vi "configure.vi"(8 "error in (no error)":errorcluster, 11 "GenericPlugin in":refnum<class "LightSourceMH110125Tsunami.lvclass">) -> (0 "error out":errorcluster, 3 "GenericPlugin out":refnum<class "LightSourceMH110125Tsunami.lvclass">)   [LabVIEW 2010, in "LightSourceMH110125Tsunami.lvclass"]
doc: "The dynamic dispatch version of this VI loads and displays the configuration file associated with the plug-in object. The user modify and save the configuration data."
uses:
  LightSourceMH110125Tsunami.lvclass
  LightSourceMH110125Tsunami.lvclass/LightSourceMH110125Tsunami.ctl
  common/classes/GenericComponent/GenericComponent/GenericComponent.lvclass
panel:
  in  "Serial port":refnum<visa-resource-name>
  in  "Switch laser on at start up?":bool caption="Switch laser on\nat start up?"
  in  "Maximal power":dbl[unit]=800.0
  in  "Read delay (ms)":u32=50
  in  "Data bits":u16=8
  in  "Baud rate":u32=9600
  in  "Parity (0:none)":enum16{"None", "Odd", "Even", "Mark", "Space"}(ring)
  in  "Stop bits":u16(ring)=10 items=["1.0"=10, "1.5"=15, "2.0"=20]
  in  "Flow control":u16(ring)=1 items=["None"=0, "XON/XOFF"=1, "RTS/CTS"=2, "DTR/DSR"=4]
  in  "cancel":bool
  in  "save":bool
  out "Configuration":string
  # "Configure MH110117Tsunami"
  # "laser settings"
  # "port settings"
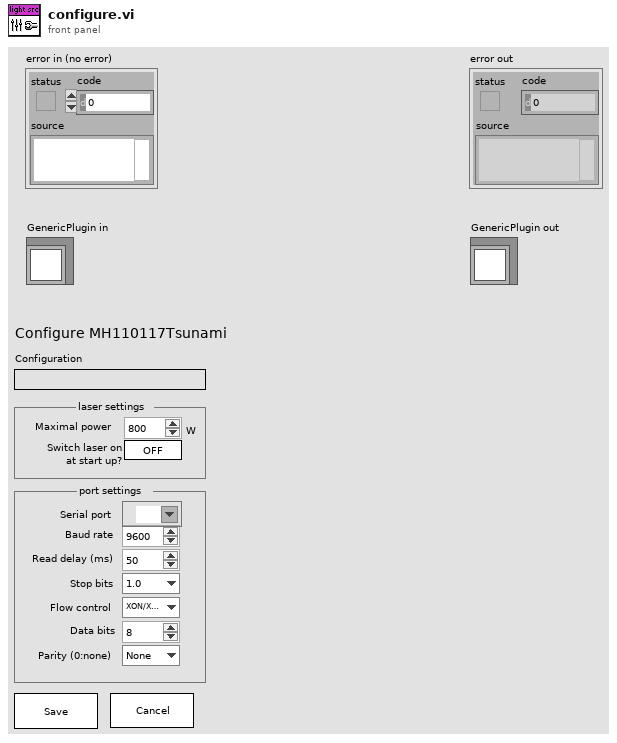
[diagram p1: front panel]
types:
  T1 = typedef "LightSourceMH110125Tsunami.lvclass/config_data_cluster.ctl" = cluster{"hardware settings":cluster{"comm port":string, "switch laser on?":bool, "open shutter?":bool, "max power":dbl[unit], "delay before read (ms)":u32, "flow control":u16, "stop bits":u16, "data bits":u16, "baud rate":u32, "parity (0:none)":enum16{"None", "Odd", "Even", "Mark", "Space"}}}
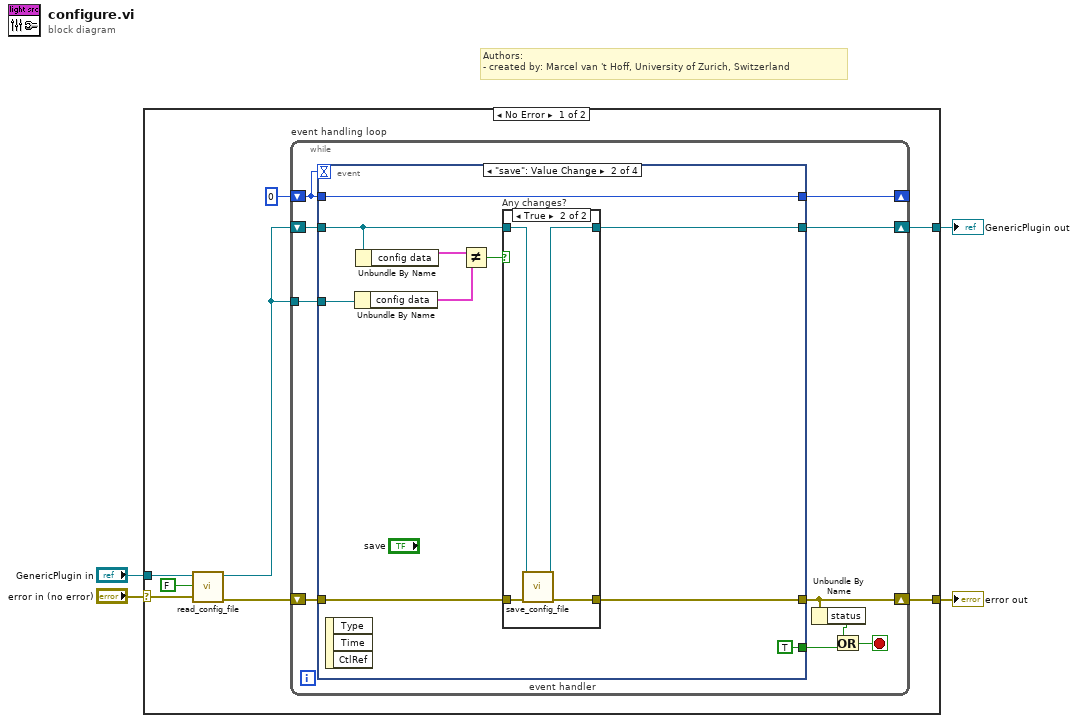
[diagram p0: block diagram]
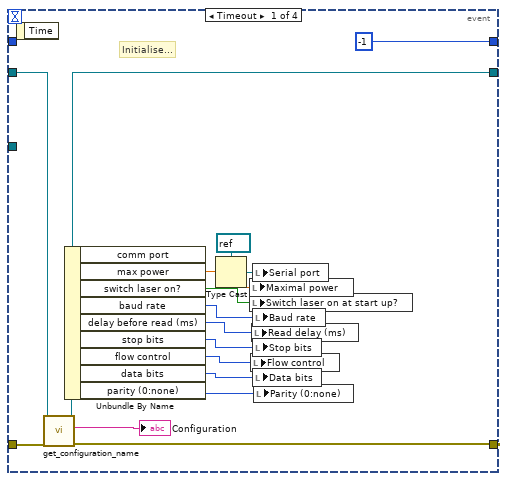
[diagram p2: hidden frame]
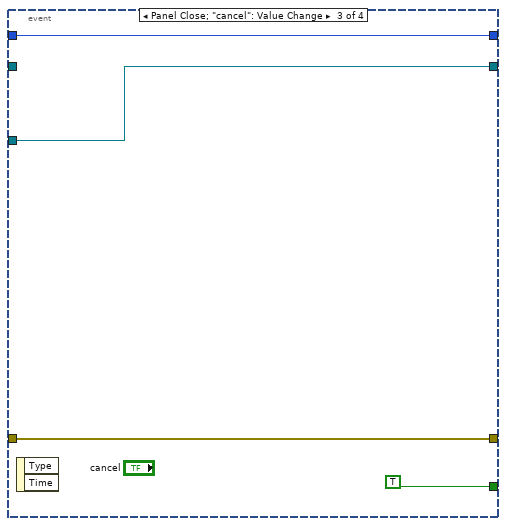
[diagram p4: hidden frame]
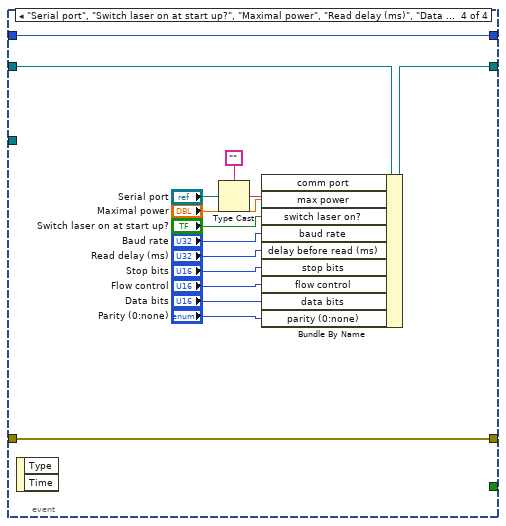
[diagram p5: hidden frame]
diagram:
  # "Authors: \n- created by: Marcel van 't Hoff, University of Zurich, Switzerland"
  n1 = case shown="No Error" "error in (no error)" {
    selector: "error in (no error)" -> [w10 w75]
    tunnel: "GenericPlugin in" -> [w8 w76]
    tunnel: [w12 w76] -> w1
    tunnel: [w11 w75] -> w2
    frame No Error {
      n2 = call-dynamic "read_config_file.vi"("error in (no error)"=w10, "force load?"=FALSE, "GenericPlugin in"=w8) -> ("error out"=w6:errorcluster, "GenericPlugin out"=w5:refnum<class "LightSourceMH110125Tsunami.lvclass">)  [unwired: 7 in]
      n3 = while "event handling loop" {
        shift-right: [w17] -> w11
        shift-left: w6 -> [w22]
        shift-right: [w20] -> w12
        shift-left: w5 -> [w21]
        shift-right: [w18] -> _
        shift-left: 0 -> [w19]
        tunnel: w5 -> [w13]
        stop <- w14 stop-if-true
        n4 = event "event handler" shown="[1] \"save\": Value Change" {
          selector: _ -> [_ _ _ _]
          dyn-events: _ -> [_ _ _ _]
          timeout: w19 -> [_ _ _ _]
          tunnel: w22 -> [w28 w47 w59 w60]
          tunnel: w21 -> [w25 w46 _ w62]
          tunnel: [w24 w43 w56 w61] -> w20
          tunnel: [w26 w44 w59 w60] -> w17
          tunnel: [_ TRUE TRUE _] -> w15
          tunnel: [-1 w48 w57 w74] -> w18
          tunnel: w19 -> [_ w48 w57 w74]
          tunnel: w13 -> [_ w41 w56 _]
          event Timeout {
            # "Initialise..."
            n5 = event-data() -> ()  [unwired: 1 in, 1 out]
            n6 = call "get_configuration_name.vi"("error in (no error)"=w28, "GenericPlugin.lvclass in"=w25) -> ("error out"=w26:errorcluster, "configuration name"=→"Configuration":string, "GenericPlugin.lvclass out"=w24:refnum<class "LightSourceMH110125Tsunami.lvclass">)  [unwired: 7 in]
            n7 = Unbundle By Name(w24) -> ("comm port"=w31:string, "max power"=w32:dbl[unit], "switch laser on?"=w33:bool, "baud rate"=w34:u32, "delay before read (ms)"=w35:u32, "stop bits"=w36:u16, "flow control"=w37:u16, "data bits"=w38:u16, "parity (0:none)"=w23:enum16{"None", "Odd", "Even", "Mark", "Space"})
            n8 = Type Cast(type=refnum<visa-resource-name> refnum ("Serial port"), x=w31) -> (*(type *) &x=w30:refnum<visa-resource-name>)
            n9 = local write "Maximal power"(w32) -> ()
            n10 = local write "Switch laser on at start up?"(w33) -> ()
            n11 = local write "Flow control"(w37) -> ()
            n12 = local write "Read delay (ms)"(w35) -> ()
            n13 = local write "Serial port"(w30) -> ()
            n14 = local write "Baud rate"(w34) -> ()
            n15 = local write "Stop bits"(w36) -> ()
            n16 = local write "Data bits"(w38) -> ()
            n17 = local write "Parity (0:none)"(w23) -> ()
          }
          event "save": Value Change {
            n18 = event-data() -> ()  [unwired: 1 in, 3 out]
            n19 = Unbundle By Name(w41) -> ("config data"=w40:T1)
            n20 = Unbundle By Name(w46) -> ("config data"=w42:T1)
            n21 = Not Equal?(x=w42, y=w40) -> (x != y?=w45:bool)
            n22 = case "Any changes?" shown="True" w45 {
              tunnel: w47 -> [w51 w54]
              tunnel: [w51 w53] -> w44
              tunnel: w46 -> [w50 w55]
              tunnel: [w50 w52] -> w43
              frame False {
              }
              frame True {
                n23 = call-dynamic "save_config_file.vi"("error in (no error)"=w54, "GenericPlugin in"=w55) -> ("error out"=w53:errorcluster, "GenericPlugin out"=w52:refnum<class "LightSourceMH110125Tsunami.lvclass">)  [unwired: 8 in]
              }
            }
          }
          event Panel Close; "cancel": Value Change {
            n24 = event-data() -> ()  [unwired: 1 in, 2 out]
          }
          event "Serial port", "Switch laser on at start up?", "Maximal power", "Read delay (ms)", "Data bits", "Baud rate", "Parity (0:none)", "Stop bits", "Flow control": Value Change {
            n25 = event-data() -> ()  [unwired: 1 in, 2 out]
            n26 = Type Cast(type="", x="Serial port") -> (*(type *) &x=w64:string)
            n27 = Bundle By Name(cluster=w62, "comm port"=w64, "max power"="Maximal power", "switch laser on?"="Switch laser on at start up?", "baud rate"="Baud rate", "delay before read (ms)"="Read delay (ms)", "stop bits"="Stop bits", "flow control"="Flow control", "data bits"="Data bits", "parity (0:none)"="Parity (0:none)") -> (w61:refnum<class "LightSourceMH110125Tsunami.lvclass">)
          }
        }
        n28 = Unbundle By Name(w17) -> ("status"=w16:bool)
        n29 = Or(x=w16, y=w15) -> (x .or. y?=w14:bool)
      }
    }
    frame Error {
    }
  }
  "error out" <- w2
  "GenericPlugin out" <- w1
